vi "SV Multitone Gain and Phase (Frequency) (1 Ch).vi"(0 "complex spectrum response":T9={"complex spectrum response"={"f0"=0.0, "df"=1.0, "complex spectrum"=[]}, "spectrum info"={"channel name"="", "description"="", "x-axis units"=0, "spectral info"={"spectrum type"=enum."Power [Magnitude^2]", "linear/dB"=enum."linear", "window"=0, "window size"=0, "FFT size"=0}, "engineering units"=0, "custom label"="", "dB reference [EU]"=0.0, "peak units"=enum."rms", "weighting filter"=0, "spectral density?"=FALSE, "unit label"="", "spectrum skewed?"=FALSE, "complimentary spectrum units"=enum."none"}} {"spectrum info"."x-axis units" items=["Time (s)"=0, "Frequency-CB (Hz)"=1, "Frequency-CPB (Hz)"=1248, "Frequency-Arbitrary (Hz)"=2357, "Quefrency (s)"=2, "Revolutions (rev)"=3, "Order"=4, "Speed (RPM)"=11, "Speed (rad/s)"=21, "Index"=65535]; "spectrum info"."weighting filter" items=["Linear", "A-weighting", "B-weighting", "C-weighting", "ITU-R 468-4", "Dolby", "CCITT", "C-message", "Wb", "Wc", "Wd", "We", "Wf", "Wh", "Wj", "Wk", "Wm", "AES17 20 kHz lowpass", "AES17 40 kHz lowpass", "AES17 20 kHz highpass", "AES17 40 kHz highpass"]; "spectrum info"."dB reference [EU]" format="%.2f"; "spectrum info"."engineering units" items=["custom..."=0, "V"=1, "A"=21, "C"=30, "pC"=31, "s"=32, "-"=29, "Pa"=2, "N"=20, "g"=3, "m/s^2"=4, "m/s"=5, "m"=6, "mm/s"=12, "mm"=13, "micron/s"=14, "micron"=15, "in/s^2"=7, "in/s"=8, "in"=9, "mil/s"=10, "mil"=11, "rad/s^2"=16, "rad/s"=17, "rad"=18, "deg/s^2"=26, "deg/s"=27, "deg"=28, "RPM"=22, "cycle/s^2"=23, "Hz"=24, "cycle"=25, "strain"=19]; "spectrum info"."spectral info"."window" items=["None "=0, "Hanning"=1, "Hamming"=2, "Blackman-Harris"=3, "Exact Blackman"=4, "Blackman"=5, "Flat Top"=6, "4 Term B-Harris "=7, "7 Term B-Harris"=8, "Low Sidelobe"=9, "Force - Exponential"=10, "Gaussian"=62]; "complex spectrum response"."complex spectrum" format="%.2f"; "complex spectrum response"."df" format="%.2f"; "complex spectrum response"."f0" format="%.2f"}, 1 "reference tones":T8(array[cluster]) {"phase (deg)" format="%0.3p"; "amplitude [EU pk]" format="%0.3p"; "frequency [Hz]" format="%0.3p"}, 5 "error in (no error)":errorcluster, 6 "desired units":T11={"gain"=enum."dB", "phase"=enum."deg", "reference level"=enum."EU rms", "response level"=enum."EU rms"}) -> (12 "unit labels":T10, 14 "complex spectrum response":T9={"complex spectrum response"={"f0"=0.0, "df"=1.0, "complex spectrum"=[]}, "spectrum info"={"channel name"="", "description"="", "x-axis units"=0, "spectral info"={"spectrum type"=enum."Power [Magnitude^2]", "linear/dB"=enum."linear", "window"=0, "window size"=0, "FFT size"=0}, "engineering units"=0, "custom label"="", "dB reference [EU]"=0.0, "peak units"=enum."rms", "weighting filter"=0, "spectral density?"=FALSE, "unit label"="", "spectrum skewed?"=FALSE, "complimentary spectrum units"=enum."none"}} {"spectrum info"."x-axis units" items=["Time (s)"=0, "Frequency-CB (Hz)"=1, "Frequency-CPB (Hz)"=1248, "Frequency-Arbitrary (Hz)"=2357, "Quefrency (s)"=2, "Revolutions (rev)"=3, "Order"=4, "Speed (RPM)"=11, "Speed (rad/s)"=21, "Index"=65535]; "spectrum info"."weighting filter" items=["Linear", "A-weighting", "B-weighting", "C-weighting", "ITU-R 468-4", "Dolby", "CCITT", "C-message", "Wb", "Wc", "Wd", "We", "Wf", "Wh", "Wj", "Wk", "Wm", "AES17 20 kHz lowpass", "AES17 40 kHz lowpass", "AES17 20 kHz highpass", "AES17 40 kHz highpass"]; "spectrum info"."dB reference [EU]" format="%.2f"; "spectrum info"."engineering units" items=["custom..."=0, "V"=1, "A"=21, "C"=30, "pC"=31, "s"=32, "-"=29, "Pa"=2, "N"=20, "g"=3, "m/s^2"=4, "m/s"=5, "m"=6, "mm/s"=12, "mm"=13, "micron/s"=14, "micron"=15, "in/s^2"=7, "in/s"=8, "in"=9, "mil/s"=10, "mil"=11, "rad/s^2"=16, "rad/s"=17, "rad"=18, "deg/s^2"=26, "deg/s"=27, "deg"=28, "RPM"=22, "cycle/s^2"=23, "Hz"=24, "cycle"=25, "strain"=19]; "spectrum info"."spectral info"."window" items=["None "=0, "Hanning"=1, "Hamming"=2, "Blackman-Harris"=3, "Exact Blackman"=4, "Blackman"=5, "Flat Top"=6, "4 Term B-Harris "=7, "7 Term B-Harris"=8, "Low Sidelobe"=9, "Force - Exponential"=10, "Gaussian"=62]; "complex spectrum response"."complex spectrum" format="%.2f"; "complex spectrum response"."df" format="%.2f"; "complex spectrum response"."f0" format="%.2f"}, 15 "gain":cluster{"frequency [Hz]":dbl[], "gain":dbl[]} {"gain" format="%_4f"; "frequency [Hz]" format="%.2f"}, 16 "phase":cluster{"frequency [Hz]":dbl[], "phase":dbl[]} {"phase" format="%.2f"; "frequency [Hz]" format="%.2f"}, 17 "gain and phase info":T1={"channel name"="", "description"="", "x-axis units"=0, "spectral info"={"spectrum type"=enum."Power [Magnitude^2]", "linear/dB"=enum."linear", "window"=0, "window size"=0, "FFT size"=0}, "engineering units"=1, "custom label"="", "dB reference [EU]"=0.0, "peak units"=enum."rms", "weighting filter"=0, "spectral density?"=FALSE, "unit label"="", "spectrum skewed?"=FALSE, "complimentary spectrum units"=enum."none"} {"x-axis units" items=["Time (s)"=0, "Frequency-CB (Hz)"=1, "Frequency-CPB (Hz)"=1248, "Frequency-Arbitrary (Hz)"=2357, "Quefrency (s)"=2, "Revolutions (rev)"=3, "Order"=4, "Speed (RPM)"=11, "Speed (rad/s)"=21, "Index"=65535]; "weighting filter" items=["Linear", "A-weighting", "B-weighting", "C-weighting", "ITU-R 468-4", "Dolby", "CCITT", "C-message", "Wb", "Wc", "Wd", "We", "Wf", "Wh", "Wj", "Wk", "Wm", "AES17 20 kHz lowpass", "AES17 40 kHz lowpass", "AES17 20 kHz highpass", "AES17 40 kHz highpass"]; "dB reference [EU]" format="%.2f"; "engineering units" items=["custom..."=0, "V"=1, "A"=21, "C"=30, "pC"=31, "s"=32, "-"=29, "Pa"=2, "N"=20, "g"=3, "m/s^2"=4, "m/s"=5, "m"=6, "mm/s"=12, "mm"=13, "micron/s"=14, "micron"=15, "in/s^2"=7, "in/s"=8, "in"=9, "mil/s"=10, "mil"=11, "rad/s^2"=16, "rad/s"=17, "rad"=18, "deg/s^2"=26, "deg/s"=27, "deg"=28, "RPM"=22, "cycle/s^2"=23, "Hz"=24, "cycle"=25, "strain"=19]; "spectral info"."window" items=["None "=0, "Hanning"=1, "Hamming"=2, "Blackman-Harris"=3, "Exact Blackman"=4, "Blackman"=5, "Flat Top"=6, "4 Term B-Harris "=7, "7 Term B-Harris"=8, "Low Sidelobe"=9, "Force - Exponential"=10, "Gaussian"=62]}, 18 "levels":T7 {"response level" format="%_6f"; "reference level" format="%_6f"}, 19 "error out":errorcluster)   [LabVIEW 2017, in "SoundVib_Multitone.lvlib"]
doc: "Use this VI to measure the gain and phase versus frequency. Wire data to <B>scaled signal [EU]</B> to determine the polymorphic instance to use or manually select the instance."
uses:
  <vilib>/addons/Sound and Vibration/svt_Multitone Distortion/SoundVib_Multitone.lvlib
  <vilib>/addons/_NISVFA/_Shared subVIs/Controls/svc_Spectrum Info.ctl
  <vilib>/addons/_NISVFA/_Shared subVIs/Controls/svc_X-Axis Units.ctl
  <vilib>/addons/_NISVFA/_Shared subVIs/Controls/svc_Spectrum Type.ctl
  <vilib>/addons/_NISVFA/_Shared subVIs/Controls/svc_Engineering Units Text Ring.ctl
  <vilib>/addons/_NISVFA/_Shared subVIs/Controls/svc_Weighting Filter Text Ring.ctl
  <vilib>/addons/_NISVFA/_Shared subVIs/Controls/svc_Complimentary Spectrum Units.ctl
  <vilib>/addons/_NISVFA/_Shared subVIs/Common/svc_Get Weighting Enum and Labels.vi
  <vilib>/addons/_NISVFA/_Shared subVIs/Common/svc_Unit Label Lexical Class.vi
  <vilib>/addons/_NISVFA/_Shared subVIs/Common/svc_Engineering Units to Unit Label.vi
  <vilib>/addons/_NISVFA/_Shared subVIs/Common/svc_Format Value (DBL).vi
  <vilib>/addons/Sound and Vibration/svt_Distortion/SoundVib_Distortion.lvlib
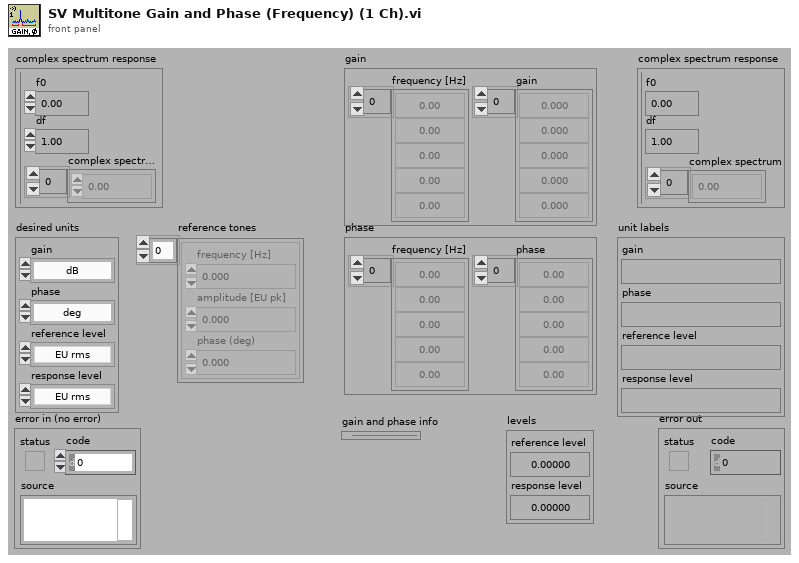
[diagram p1: front panel]
types:
  T1 = typedef "svc_Spectrum Info.ctl" = cluster{"channel name":string, "description":string, "x-axis units":T2, "spectral info":cluster{"spectrum type":T3, "linear/dB":enum16{"linear", "dB"}, "window":u16, "window size":i32, "FFT size":i32}, "engineering units":T4, "custom label":string, "dB reference [EU]":dbl, "peak units":enum16{"rms", "peak", "peak-peak"}, "weighting filter":T5, "spectral density?":bool, "unit label":string, "spectrum skewed?":bool, "complimentary spectrum units":T6}
  T2 = typedef "svc_X-Axis Units.ctl" = u16
  T3 = typedef "svc_Spectrum Type.ctl" = enum16{"FFT Spectrum [complex]", "Amplitude [Magnitude]", "Power [Magnitude^2]", "Cross Spectrum [complex]", "Frequency Response [Complex]"}
  T4 = typedef "svc_Engineering Units Text Ring.ctl" = u16
  T5 = typedef "svc_Weighting Filter Text Ring.ctl" = u16
  T6 = typedef "svc_Complimentary Spectrum Units.ctl" = enum16{"none", "radians", "degrees", "cycles", "imaginary"}
  T7 = cluster{"reference level":dbl, "response level":dbl}
  T8 = cluster{"frequency [Hz]":dbl, "amplitude [EU pk]":dbl, "phase (deg)":dbl}[]
  T9 = cluster{"complex spectrum response":cluster{"f0":dbl, "df":dbl, "complex spectrum":cdb[]}, "spectrum info":T1}
  T10 = cluster{"gain":string, "phase":string, "reference level":string, "response level":string}
  T11 = cluster{"gain":enum16{"dB", "linear ratio", "%"}, "phase":enum16{"deg", "rad"}, "reference level":enum16{"EU^2 rms", "EU rms", "dB", "dBc", "dBV", "dBu", "dBm"}, "response level":enum16{"EU^2 rms", "EU rms", "dB", "dBc", "dBV", "dBu", "dBm"}}
  T12 = enum16{"No change", "Unwrap", "Wrap: -360 to 0", "Wrap: -270 to 90", "Wrap: -180 to 180", "Wrap: -90 to 270", "Wrap: 0 to 360", "Wrap: custom range"}
  T13 = cluster{"frequency [Hz]":dbl, "amplitude [EU pk]":dbl, "phase [deg]":dbl}
  T14 = enum16{"EU^2 rms", "EU rms", "dB", "dBc", "dBV", "dBu", "dBm"}
  T15 = cluster{"converted level":dbl, "converted level":dbl}
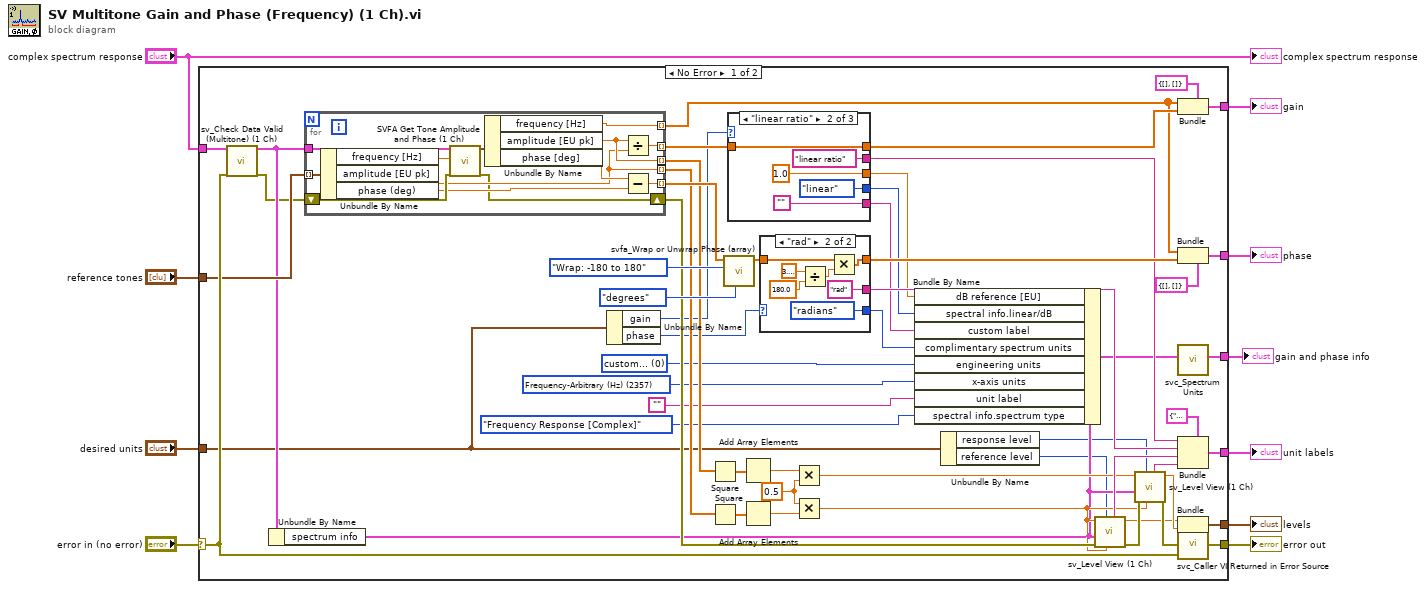
[diagram p0: block diagram]
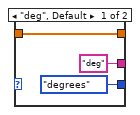
[diagram p2: hidden frame]
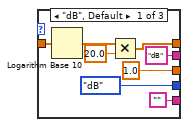
[diagram p3: hidden frame]
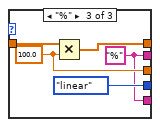
[diagram p4: hidden frame]
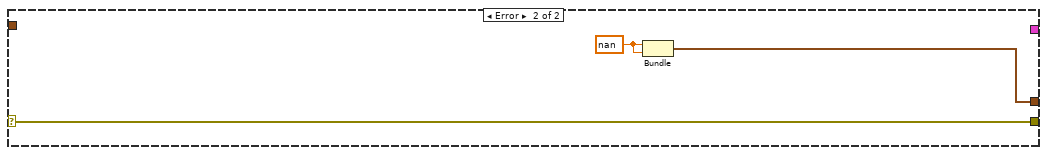
[diagram p5: hidden frame]
diagram:
  n1 = case shown="No Error" "error in (no error)" {
    selector: "error in (no error)" -> [w62 w109]
    tunnel: "complex spectrum response" -> [w63 _]
    tunnel: [w65 w109] -> w9
    tunnel: "desired units" -> [w15 _]
    tunnel: [w64 _] -> w6
    tunnel: "reference tones" -> [w61 _]
    tunnel: [w44 _] -> w4
    tunnel: [w43 _] -> w3
    tunnel: [w32 w107] -> w2
    tunnel: [w14 _] -> w1
    frame No Error {
      w25 = T2 2357 items=["Time (s)"=0, "Frequency-CB (Hz)"=1, "Frequency-CPB (Hz)"=1248, "Frequency-Arbitrary (Hz)"=2357, "Quefrency (s)"=2, "Revolutions (rev)"=3, "Order"=4, "Speed (RPM)"=11, "Speed (rad/s)"=21, "Critical Band"=31, "Critical Band Rate (Bark)"=32, "Index"=65535] ("x-axis units")
      w21 = T4 0 items=["custom..."=0, "V"=1, "A"=21, "Pa"=2, "N"=20, "g"=3, "m/s^2"=4, "m/s"=5, "m"=6, "mm/s"=12, "mm"=13, "micron/s"=14, "micron"=15, "in/s^2"=7, "in/s"=8, "in"=9, "mil/s"=10, "mil"=11, "rad/s^2"=16, "rad/s"=17, "rad"=18, "deg/s^2"=26, "deg/s"=27, "deg"=28, "RPM"=22, "cycle/s^2"=23, "Hz"=24, "cycle"=25, "strain"=19] ("engineering units")
      w35 = 0.5 ("y")
      n2 = call <vilib>:"sv_Check Data Valid (Multitone) (1 Ch).vi"("complex spectrum"=w63, "error in (no error)"=w62) -> ("complex spectrum"=w60:T9, "error out"=w31:errorcluster)  [unwired: 15 in, 1 out]
      n3 = Unbundle By Name(w60) -> ("spectrum info"=w28:T1)
      n4 = for {
        tunnel: w61 -> [w105] mode=indexing
        tunnel: w60 -> [w106]
        tunnel: [w100] -> w59 mode=indexing
        tunnel: [w99] -> w57 mode=indexing
        tunnel: [w98] -> w54 mode=indexing
        tunnel: [w97] -> w51 mode=indexing
        shift-right: [w96] -> w39
        shift-left: w31 -> [w103]
        tunnel: [w94] -> w42 mode=indexing
        n5 = Unbundle By Name(w105) -> ("frequency [Hz]"=w95:dbl, "amplitude [EU pk]"=w97:dbl, "phase (deg)"=w101:dbl)
        n6 = call <vilib>:"SVFA Get Tone Amplitude and Phase (1 Ch).vi"("complex spectrum"=w106, "tone frequency [Hz]"=w95, "error in (no error)"=w103) -> ("identified tone"=w104:T13, "error out"=w96:errorcluster)  [unwired: 15 in]
        n7 = Unbundle By Name(w104) -> ("frequency [Hz]"=w94:dbl, "amplitude [EU pk]"=w98:dbl, "phase [deg]"=w102:dbl)
        n8 = Divide(x=w98, y=w97) -> (x/y=w100:dbl)
        n9 = Subtract(x=w102, y=w101) -> (x-y=w99:dbl)
      }
      n10 = Unbundle By Name(w15) -> ("gain"=w30:enum16{"dB", "linear ratio", "%"}, "phase"=w29:enum16{"deg", "rad"})
      n11 = Square(x=w54) -> (x^2=w53:dbl[])
      n12 = Square(x=w51) -> (x^2=w52:dbl[])
      n13 = call <vilib>:"svfa_Wrap or Unwrap Phase (array).vi"("phase units"=svc_Complimentary_Spectrum_Units."degrees", "desired wrapping"=T12."Wrap: -180 to 180", "phase in"=w57) -> ("phase out"=w55:dbl[])  [unwired: 7 in, 1 out]
      n14 = case shown="\"linear ratio\"" w30 {
        tunnel: [w80 w88 w92] -> w46
        tunnel: w59 -> [w83 w88 w93]
        tunnel: ["dB" "linear ratio" w89] -> w27
        tunnel: [1.0 ("y") 1.0 ("y") w91] -> w20
        tunnel: [enum16{"linear", "dB"}."dB" ("linear/dB") enum16{"linear", "dB"}."linear" ("linear/dB") enum16{"linear", "dB"}."linear" ("linear/dB")] -> w19
        tunnel: ["" "" w89] -> w18
        frame "dB", Default {
          n15 = Logarithm Base 10(1:w83) -> (0:w82:dbl[])
          n16 = Multiply(x=w82, y=20.0) -> (x*y=w80:dbl[])
        }
        frame "linear ratio" {
        }
        frame "%" {
          w89 = "%"
          w91 = 100.0 ("y")
          n17 = Multiply(x=w93, y=w91) -> (x*y=w92:dbl[])
        }
      }
      n18 = Add Array Elements(numeric array=w53) -> (sum=w50:dbl)
      n19 = Add Array Elements(numeric array=w52) -> (sum=w37:dbl)
      n20 = case shown="\"rad\"" w29 {
        tunnel: w55 -> [w68 w73]
        tunnel: [w68 w71] -> w45
        tunnel: ["deg" "rad"] -> w47
        tunnel: [svc_Complimentary_Spectrum_Units."degrees" ("complimentary spectrum units") svc_Complimentary_Spectrum_Units."radians" ("complimentary spectrum units")] -> w26
        frame "deg", Default {
        }
        frame "rad" {
          n21 = Divide(x=3.141592653589793, y=180.0) -> (x/y=w72:dbl)
          n22 = Multiply(x=w73, y=w72) -> (x*y=w71:dbl[])
        }
      }
      n23 = Multiply(x=w50, y=w35) -> (x*y=w38:dbl)
      n24 = Multiply(x=w35, y=w37) -> (x*y=w36:dbl)
      n25 = Bundle By Name(cluster=w28, "dB reference [EU]"=w20, "spectral info.linear/dB"=w19, "custom label"=w18, "complimentary spectrum units"=w26, "engineering units"=w21, "x-axis units"=w25, "unit label"="", "spectral info.spectrum type"=svc_Spectrum_Type."Frequency Response [Complex]" ("spectrum type")) -> (w22:T1)
      n26 = Unbundle By Name(w15) -> ("response level"=w17:T14, "reference level"=w16:T14)
      n27 = call <vilib>:"sv_Level View (1 Ch).vi"("carrier level [EU^2 rms]"=w36, "desired units"=w16, "error in (no error)"=w39, "spectrum info"=w28, "level [EU^2 rms]"=w36) -> ("error out"=w41:errorcluster, "converted level"=w33:dbl, "unit label"=w49:string)  [unwired: 4 in]
      n28 = call <vilib>:"sv_Level View (1 Ch).vi"("carrier level [EU^2 rms]"=w36, "desired units"=w17, "error in (no error)"=w41, "spectrum info"=w28, "level [EU^2 rms]"=w38) -> ("error out"=w40:errorcluster, "converted level"=w34:dbl, "unit label"=w48:string)  [unwired: 4 in]
      n29 = Bundle(cluster=cluster{"frequency [Hz]":dbl[], "gain":dbl[]} {"frequency [Hz]"=[], "gain"=[]} ("gain"), "frequency [Hz]"=w42, "gain"=w46) -> (w43:cluster{"frequency [Hz]":dbl[], "gain":dbl[]})
      n30 = Bundle(cluster=cluster{"frequency [Hz]":dbl[], "phase":dbl[]} {"frequency [Hz]"=[], "phase"=[]} ("phase"), "frequency [Hz]"=w42, "phase"=w45) -> (w44:cluster{"frequency [Hz]":dbl[], "phase":dbl[]})
      n31 = call <vilib>:"svc_Spectrum Units.vi"("spectrum info in"=w22) -> ("spectrum info out"=w14:T1)  [unwired: 3 in, 3 out]
      n32 = Bundle(cluster=T10 {"gain"="", "phase"="", "reference level"="", "response level"=""} ("unit labels"), "gain"=w27, "phase"=w47, "reference level"=w49, "response level"=w48) -> (w64:T10)
      n33 = Bundle("converted level"=w33, "converted level"=w34) -> (w32:T15)  [unwired: 1 in]
      n34 = call <vilib>:"svc_Caller VI Returned in Error Source.vi"("warning input to caller"=w62, "error in (no error)"=w40) -> ("error out"=w65:errorcluster)  [unwired: 3 in]
    }
    frame Error {
      w108 = nan ("SINAD")
      n35 = Bundle("SINAD"=w108, "SINAD"=w108) -> (w107:cluster{"SINAD":dbl, "SINAD":dbl})  [unwired: 1 in]
    }
  }
  "error out" <- w9
  "phase" <- w4
  "unit labels" <- w6
  "gain" <- w3
  "levels" <- w2
  "gain and phase info" <- w1
  "complex spectrum response" <- "complex spectrum response"
